vi "PIDController_SetI.vi"(9 "Ki":dbl, 11 "in PID_CONTROLLER":T1={"Kp"=0.0, "Ki"=0.0, "Kd"=0.0, "Period"=0.0, "Max_Integral"=0.0, "Min_Integral"=0.0, "Max_Input"=0.0, "Min_Input"=0.0, "Input_Range"=0.0, "Continuous"=FALSE, "PositionError"=0.0, "VelocityError"=0.0, "PrevError"=0.0, "TotalError"=0.0, "PositionTolerance"=0.0, "VelocityTolerance"=0.0, "SetPoint"=0.0, "Kf"=0.0, "Prev_Deriv"=0.0, "Prev_Deriv 2"=0.0, "DerivativeFilter"=FALSE, "Min_Output"=-9.99e+35, "Max_Output"=9.9e+35, "Prev_F_P"=0.0, "Prev_F_P_2"=0.0, "AntiWindupActive"=FALSE} {"Prev_F_P_2" format="%16_6e"; "Prev_F_P" format="%16_6e"; "Max_Output" format="%16_6e"; "Min_Output" format="%16_6e"; "Prev_Deriv 2" format="%16_6e"; "Prev_Deriv" format="%16_6e"; "Kf" format="%16_6e"; "SetPoint" format="%17.6f"; "VelocityTolerance" format="%17.6f"; "PositionTolerance" format="%17.6f"; "TotalError" format="%17.6f"; "PrevError" format="%17.6f"; "VelocityError" format="%17.6f"; "PositionError" format="%17.6f"; "Input_Range" format="%17.6f"; "Min_Input" format="%17.6f"; "Max_Input" format="%17.6f"; "Min_Integral" format="%17.6f"; "Max_Integral" format="%17.6f"; "Period" format="%17.6f"; "Kd" format="%17.6f"; "Ki" format="%17.6f"; "Kp" format="%17.6f"}) -> (3 "out PID_CONTROLLER":T1={"Kp"=0.0, "Ki"=0.0, "Kd"=0.0, "Period"=0.0, "Max_Integral"=0.0, "Min_Integral"=0.0, "Max_Input"=0.0, "Min_Input"=0.0, "Input_Range"=0.0, "Continuous"=FALSE, "PositionError"=0.0, "VelocityError"=0.0, "PrevError"=0.0, "TotalError"=0.0, "PositionTolerance"=0.0, "VelocityTolerance"=0.0, "SetPoint"=0.0, "Kf"=0.0, "Prev_Deriv"=0.0, "Prev_Deriv 2"=0.0, "DerivativeFilter"=FALSE, "Min_Output"=-9.99e+35, "Max_Output"=9.9e+35, "Prev_F_P"=0.0, "Prev_F_P_2"=0.0, "AntiWindupActive"=FALSE} {"Prev_F_P_2" format="%16_6e"; "Prev_F_P" format="%16_6e"; "Max_Output" format="%16_6e"; "Min_Output" format="%16_6e"; "Prev_Deriv 2" format="%16_6e"; "Prev_Deriv" format="%16_6e"; "Kf" format="%16_6e"; "SetPoint" format="%17.6f"; "VelocityTolerance" format="%17.6f"; "PositionTolerance" format="%17.6f"; "TotalError" format="%17.6f"; "PrevError" format="%17.6f"; "VelocityError" format="%17.6f"; "PositionError" format="%17.6f"; "Input_Range" format="%17.6f"; "Min_Input" format="%17.6f"; "Max_Input" format="%17.6f"; "Min_Integral" format="%17.6f"; "Max_Integral" format="%17.6f"; "Period" format="%17.6f"; "Kd" format="%17.6f"; "Ki" format="%17.6f"; "Kp" format="%17.6f"})   [LabVIEW 2019, in "Trajectory_Library.lvlib"]
doc: "Sets the Integral coefficient of the PID controller gain.\n \nInputs:\n - PID_Controller -- PID_Controller data cluster\n - Ki -- integral coefficient\n\nOutputs:\n - PID_Controller -- Updated PID_Controller data cluster"
uses:
  Trajectory_Library.lvlib
  PID_CONTROLLER.ctl
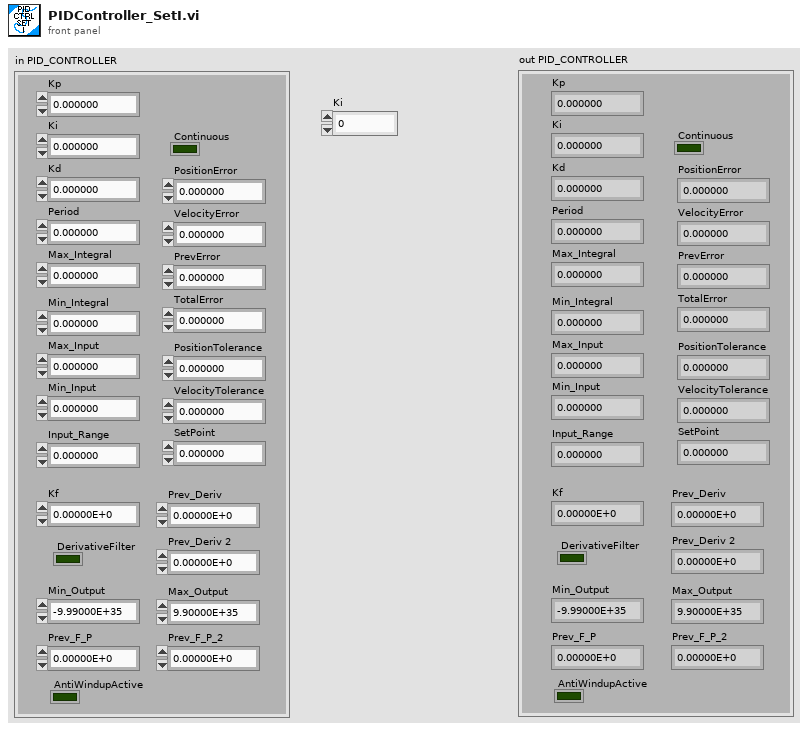
[diagram p1: front panel]
types:
  T1 = typedef "Trajectory_Library.lvlib/PID_CONTROLLER.ctl" = cluster{"Kp":dbl, "Ki":dbl, "Kd":dbl, "Period":dbl, "Max_Integral":dbl, "Min_Integral":dbl, "Max_Input":dbl, "Min_Input":dbl, "Input_Range":dbl, "Continuous":bool, "PositionError":dbl, "VelocityError":dbl, "PrevError":dbl, "TotalError":dbl, "PositionTolerance":dbl, "VelocityTolerance":dbl, "SetPoint":dbl, "Kf":dbl, "Prev_Deriv":dbl, "Prev_Deriv 2":dbl, "DerivativeFilter":bool, "Min_Output":dbl, "Max_Output":dbl, "Prev_F_P":dbl, "Prev_F_P_2":dbl, "AntiWindupActive":bool}
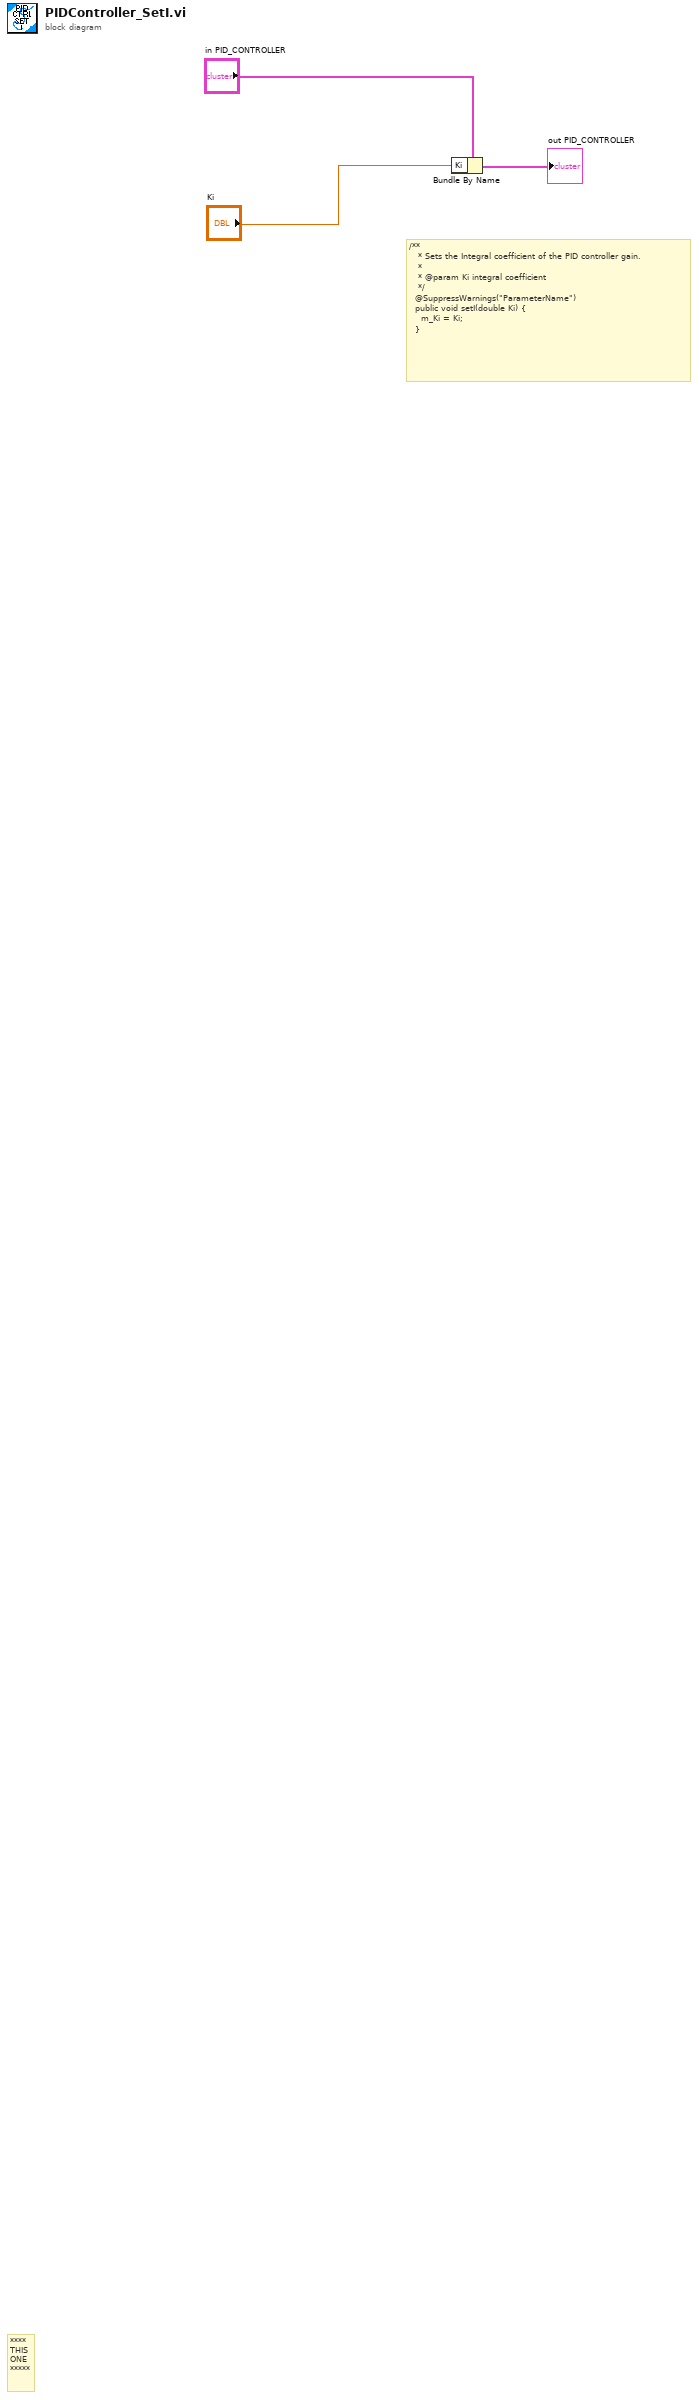
[diagram p0: block diagram]
diagram:
  # "/**\n   * Sets the Integral coefficient of the PID controller gain.\n   *\n   * @param Ki integral coefficient\n   */\n  @SuppressWarnings(\"ParameterName\")\n  public void setI(double Ki) {\n    m_Ki = Ki;\n  }"
  # "****\nTHIS\nONE\n*****"
  n1 = Bundle By Name(cluster="in PID_CONTROLLER", "Ki"="Ki") -> (→"out PID_CONTROLLER":T1)
